vi "Given When Then.vi"   [LabVIEW 2015]
doc: "Provides a standard Given, When, Then structure for tests.\n\nDesigned to drop and fill the standard VI tester template."
uses:
  <vilib>/addons/_JKI Toolkits/VI Tester/TestCase.llb/TestCase.lvclass
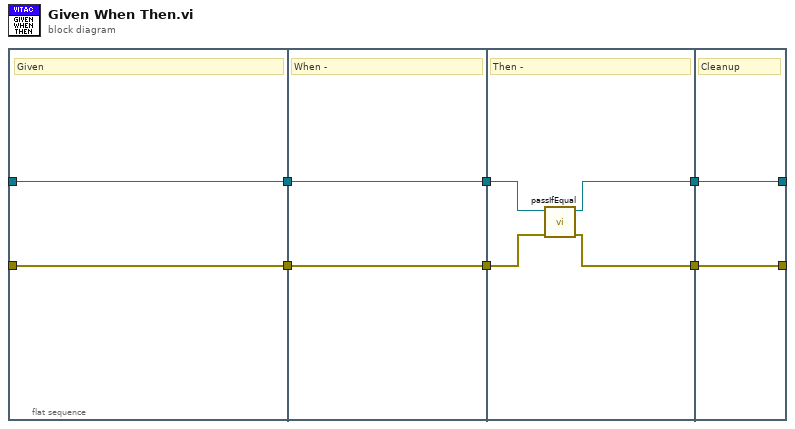
[diagram p0: block diagram]
diagram:
  n1 = flat-sequence {
    tunnel: _ -> [w7]
    tunnel: _ -> [w8]
    tunnel: [w8] -> w6
    tunnel: [w7] -> w5
    tunnel: [w10] -> w4
    tunnel: [w9] -> w3
    tunnel: w6 -> [w10]
    tunnel: w5 -> [w9]
    tunnel: [w13] -> w2
    tunnel: [w11] -> w1
    tunnel: w4 -> [w14]
    tunnel: w3 -> [w12]
    tunnel: [w15] -> _
    tunnel: [w16] -> _
    tunnel: w2 -> [w16]
    tunnel: w1 -> [w15]
    frame #0 {
      # "Given"
    }
    frame #1 {
      # "When -"
    }
    frame #2 {
      # "Then -"
      n2 = call-dynamic "passIfEqual.vi"("error in (no error)"=w12, "TestCase in"=w14) -> ("error out"=w11:errorcluster, "TestCase out"=w13:refnum<class "TestCase.lvclass">)  [unwired: 8 in]
    }
    frame #3 {
      # "Cleanup"
    }
  }
